vi "Vision Processing.vi"(4 "error in (no error)":errorcluster) -> ()   [LabVIEW 2014]
doc: "This VI runs in parallel to other tasks. It gets images from the camera, processes them for color or shape and use that information to affect robot behavior."
uses:
  <vilib>/Rock Robotics/WPI/Camera/WPI_CameraWhite Balance Values.ctl
  <vilib>/Rock Robotics/WPI/Camera/WPI_CameraExposure Values.ctl
  <vilib>/Rock Robotics/WPI/Camera/WPI_CameraFrameRate.ctl
  <vilib>/Rock Robotics/WPI/Camera/WPI_CameraImageSize.ctl
  Robot Global Data.vi
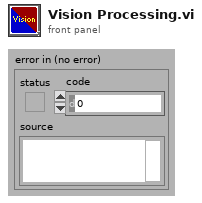
[diagram p1: front panel]
types:
  T1 = typedef "WPI_CameraImageSize.ctl" = enum16{"640x480", "320x240", "160x120", "Custom"}
  T2 = typedef "WPI_CameraFrameRate.ctl" = u32
  T3 = typedef "WPI_CameraExposure Values.ctl" = enum16{"Auto", "Flicker-free 50 Hz", "Flicker-free 60 Hz", "Hold current", "Custom"}
  T4 = typedef "WPI_CameraWhite Balance Values.ctl" = enum16{"Auto", "Fixed indoor", "Fixed outdoor 1", "Fixed outdoor 2", "Fixed fluorescent 1", "Fixed fluorescent 2", "Hold current", "Custom"}
  T5 = typedef "Image Type" = u32
  T6 = typedef "WPI_CameraDevRef.ctl" = cluster{"Camera Address":string, "CameraStatus":errorcluster}
  T7 = typedef "IMAQ Image.ctl" = refnum<image>
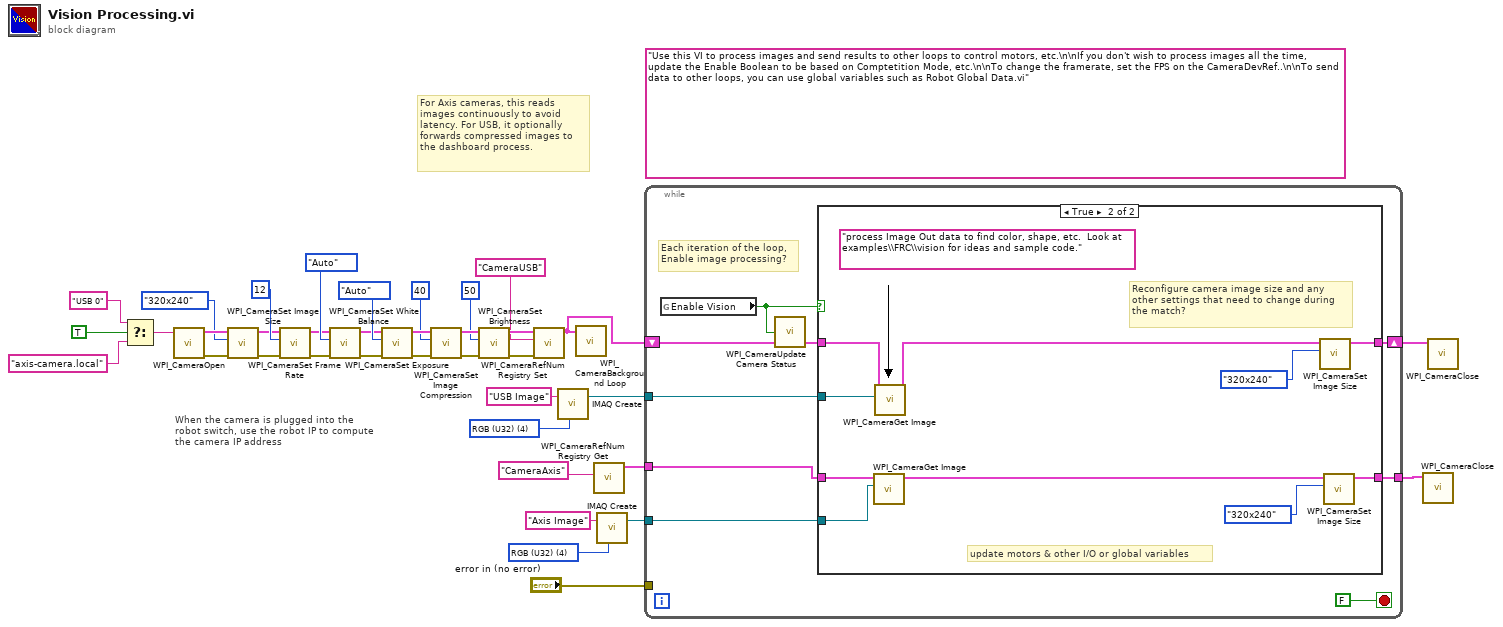
[diagram p0: block diagram]
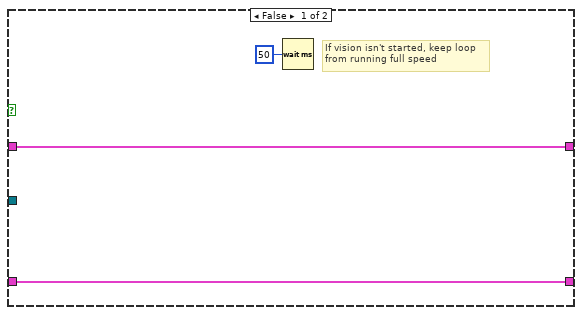
[diagram p2: hidden frame]
diagram:
  w30 = T5 4 items=["Grayscale (U8)", "Grayscale (I16)", "Grayscale (SGL)", "Complex (CSG)", "RGB (U32)", "HSL (U32)", "RGB (U64)"] ("Image Type")
  (unwired) "Use this VI to process images and send results to other loops to control motors, etc.\n\nIf you don't wish to process images all the time, update the Enable Boolean to be based on Comptetition Mode, etc.\n\nTo change the framerate, set the FPS on the CameraDevRef..\n\nTo send data to other loops, you can use global variables such as Robot Global Data.vi"
  w37 = T5 4 items=["Grayscale (U8)", "Grayscale (I16)", "Grayscale (SGL)", "Complex (CSG)", "RGB (U32)", "HSL (U32)", "RGB (U64)"] ("Image Type")
  # "When the camera is plugged into the\nrobot switch, use the robot IP to compute\nthe camera IP address"
  # "For Axis cameras, this reads\nimages continuously to avoid\nlatency. For USB, it optionally\nforwards compressed images to\nthe dashboard process."
  n1 = Select(t="USB 0" ("format string"), s=TRUE ("dot notation? (F)"), f="axis-camera.local" ("format string")) -> (s? t:f=w25:string)
  n2 = call <vilib>:"WPI_CameraOpen.vi"("Camera Address"=w25) -> ("error out"=w12:errorcluster, "CameraDevRef"=w11:T6)  [unwired: 1 in, 8 out]
  n3 = call <vilib>:"WPI_CameraSet Image Size.vi"("error in (no error)"=w12, "Image Size"=WPI_CameraImageSize."320x240", "CameraDevRef"=w11) -> ("error out"=w13:errorcluster, "CameraDevRef Out"=w10:T6)  [unwired: 1 in, 6 out]
  n4 = call <vilib>:"WPI_CameraSet Frame Rate.vi"("error in (no error)"=w13, "Frame Rate (fps)"=T2 12, "CameraDevRef"=w10) -> ("error out"=w14:errorcluster, "CameraDevRef Out"=w8:T6)  [unwired: 7 out]
  n5 = call <vilib>:"WPI_CameraSet White Balance.vi"("error in (no error)"=w14, "White Balance"=WPI_CameraWhite_Balance_Values."Auto", "CameraDevRef"=w8) -> ("error out"=w15:errorcluster, "CameraDevRef Out"=w9:T6)  [unwired: 1 in, 6 out]
  n6 = call <vilib>:"WPI_CameraSet Exposure.vi"("error in (no error)"=w15, "Exposure"=WPI_CameraExposure_Values."Auto", "CameraDevRef"=w9) -> ("error out"=w16:errorcluster, "CameraDevRef Out"=w6:T6)  [unwired: 1 in, 6 out]
  n7 = call <vilib>:"WPI_CameraSet Image Compression.vi"("error in (no error)"=w16, "Compression"=40, "CameraDevRef"=w6) -> ("error out"=w17:errorcluster, "CameraDevRef Out"=w7:T6)  [unwired: 7 out]
  n8 = call <vilib>:"WPI_CameraSet Brightness.vi"("error in (no error)"=w17, "Brightness"=50, "CameraDevRef"=w7) -> ("error out"=w19:errorcluster, "CameraDevRef Out"=w18:T6)  [unwired: 7 out]
  n9 = call <vilib>:"WPI_CameraRefNum Registry Set.vi"("error in (no error)"=w19, "refnum name"="CameraUSB", "CameraDevRef"=w18) -> ("CameraDevRef"=w1:T6)  [unwired: 8 out]
  n10 = call "IMAQ Create"("Image Name"="USB Image", "Image Type"=w37) -> ("New Image"=w35:T7)  [unwired: 2 in, 2 out]
  n11 = call <vilib>:"WPI_CameraBackground Loop.vi"("CameraDevRef"=w1) -> ()  [unwired: 11 in]
  n12 = call <vilib>:"WPI_CameraRefNum Registry Get.vi"("refnum name"="CameraAxis") -> ("CameraDevRef"=w29:T6)  [unwired: 9 in, 1 out]
  n13 = call "IMAQ Create"("Image Name"="Axis Image", "Image Type"=w30) -> ("New Image"=w28:T7)  [unwired: 2 in, 2 out]
  n14 = while {
    shift-right: [w45] -> w34
    shift-left: w1 -> [w43]
    tunnel: w35 -> [w44]
    tunnel: "error in (no error)" -> [_]
    tunnel: w29 -> [w38]
    tunnel: w28 -> [w40]
    tunnel: [w39] -> w27
    stop <- FALSE stop-if-true
    # "Each iteration of the loop,\nEnable image processing?"
    n15 = global read "Robot Global Data.vi" "Enable Vision"() -> (w41:bool)
    n16 = call <vilib>:"WPI_CameraUpdate Camera Status.vi"("CameraDevRef In"=w43, "Enable Vision"=w41) -> ("CameraDevRef Out"=w42:T6)  [unwired: 3 in]
    n17 = case shown="True" w41 {
      tunnel: w44 -> [_ w58]
      tunnel: [w49 w59] -> w45
      tunnel: w42 -> [w49 w57]
      tunnel: w38 -> [w47 w54]
      tunnel: w40 -> [_ w53]
      tunnel: [w47 w50] -> w39
      frame False {
        # "If vision isn't started, keep loop\nfrom running full speed"
        n18 = Wait (ms)(milliseconds to wait=u32 50) -> ()  [unwired: 1 out]
      }
      frame True {
        (unwired) "process Image Out data to find color, shape, etc.  Look at examples\\FRC\\vision for ideas and sample code."
        # "update motors & other I/O or global variables"
        # "Reconfigure camera image size and any\nother settings that need to change during\nthe match?"
        n19 = call <vilib>:"WPI_CameraGet Image.vi"("Image"=w53, "CameraDevRef"=w54) -> ("CameraDevRef Out"=w51:T6)  [unwired: 1 in, 8 out]
        n20 = call <vilib>:"WPI_CameraGet Image.vi"("Image"=w58, "CameraDevRef"=w57) -> ("CameraDevRef Out"=w56:T6)  [unwired: 1 in, 8 out]
        n21 = call <vilib>:"WPI_CameraSet Image Size.vi"("Image Size"=WPI_CameraImageSize."320x240", "CameraDevRef"=w56) -> ("CameraDevRef Out"=w59:T6)  [unwired: 2 in, 7 out]
        n22 = call <vilib>:"WPI_CameraSet Image Size.vi"("Image Size"=WPI_CameraImageSize."320x240", "CameraDevRef"=w51) -> ("CameraDevRef Out"=w50:T6)  [unwired: 2 in, 7 out]
      }
    }
  }
  n23 = call <vilib>:"WPI_CameraClose.vi"("CameraDevRef"=w27) -> ()  [unwired: 1 in, 10 out]
  n24 = call <vilib>:"WPI_CameraClose.vi"("CameraDevRef"=w34) -> ()  [unwired: 1 in, 10 out]
